vi "Send On Event Message.vi"(8 "error in (no error)":errorcluster, 10 "Event":string, 11 "Observable Actor in":refnum<class "Observable Actor.lvclass">) -> (0 "error out":errorcluster, 3 "Observable Actor out":refnum<class "Observable Actor.lvclass">)   [LabVIEW 2014, in "Observable Actor.lvlib" / "Observable Actor.lvclass"]
uses:
  Observable Actor.lvclass
  Observable Actor.lvclass/Observable Actor.ctl
  <vilib>/ActorFramework/Message Enqueuer/Message Enqueuer.lvclass/Message Enqueuer.ctl
  <vilib>/ActorFramework/Message Priority Queue/Priority Enqueue.vi
  <vilib>/ActorFramework/Message Enqueuer/Message Enqueuer.lvclass
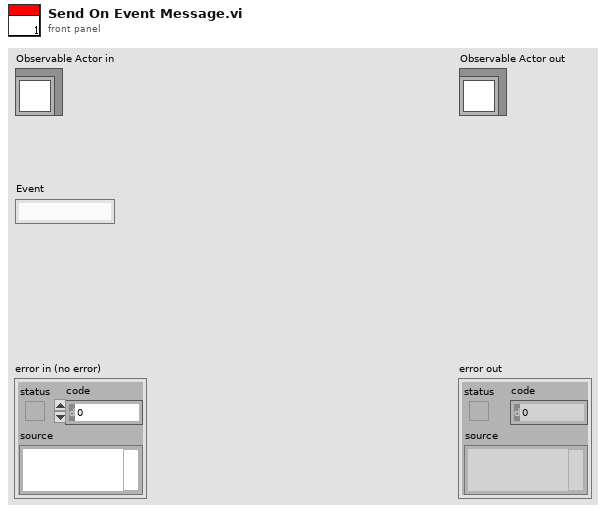
[diagram p1: front panel]
types:
  T1 = typedef "MessageToSend.ctl" = cluster{"Enqueuer":refnum<class "Message Enqueuer.lvclass">, "Message":refnum<class "Message.lvclass">}
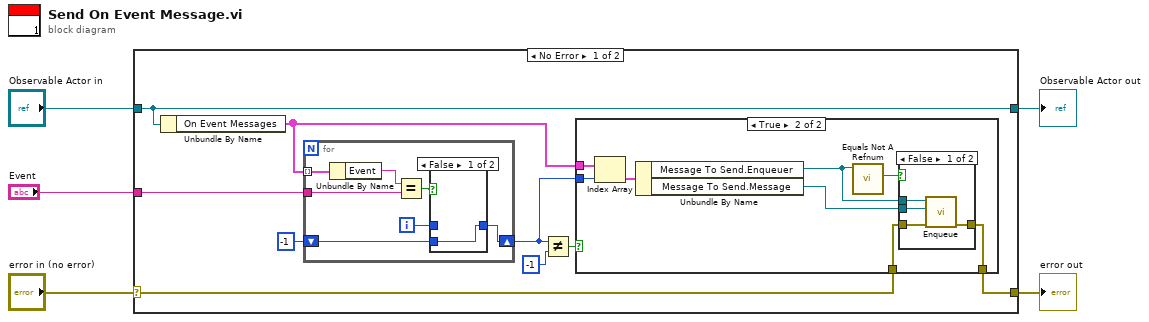
[diagram p0: block diagram]
diagram:
  n1 = case shown="No Error" "error in (no error)" {
    selector: "error in (no error)" -> [w7 w39]
    tunnel: [w6 w39] -> w4
    tunnel: [w14 w38] -> w2
    tunnel: "Observable Actor in" -> [w14 w38]
    tunnel: "Event" -> [w13 _]
    frame No Error {
      n2 = Unbundle By Name(w14) -> ("On Event Messages"=w9:cluster{"Event":string, "Message To Send":T1}[])
      n3 = for {
        tunnel: w9 -> [w35] mode=indexing
        tunnel: w13 -> [w32]
        shift-right: [w30] -> w8
        shift-left: -1 -> [w29]
        i -> [w31]
        n4 = Unbundle By Name(w35) -> ("Event"=w33:string)
        n5 = Equal?(x=w33, y=w32) -> (x = y?=w34:bool)
        n6 = case shown="False" w34 {
          tunnel: w31 -> [_ w37]
          tunnel: [w36 w37] -> w30
          tunnel: w29 -> [w36 _]
          frame False {
          }
          frame True {
          }
        }
      }
      n7 = Not Equal?(x=w8, y=-1) -> (x != y?=w10:bool)
      n8 = case shown="True" w10 {
        tunnel: w9 -> [_ w23]
        tunnel: w8 -> [_ w22]
        tunnel: w7 -> [w15 w17]
        tunnel: [w15 w16] -> w6
        frame False {
        }
        frame True {
          n9 = Index Array(array=w23, index=w22) -> (element=w21:cluster{"Event":string, "Message To Send":T1})
          n10 = Unbundle By Name(w21) -> ("Message To Send.Enqueuer"=w19:refnum<class "Message Enqueuer.lvclass">, "Message To Send.Message"=w18:refnum<class "Message.lvclass">)
          n11 = call <vilib>:"Equals Not A Refnum.vi"("Message Enqueuer"=w19) -> ("Not a refnum?"=w20:bool)  [unwired: 10 in]
          n12 = case shown="False" w20 {
            tunnel: w18 -> [w26 _]
            tunnel: w19 -> [w27 _]
            tunnel: w17 -> [w25 w28]
            tunnel: [w24 w28] -> w16
            frame False {
              n13 = call <vilib>:"Enqueue.vi"("error in (no error)"=w25, "Message"=w26, "Message Enqueuer in"=w27) -> ("error out"=w24:errorcluster)  [unwired: 7 in, 1 out]
            }
            frame True {
            }
          }
        }
      }
    }
    frame Error {
    }
  }
  "error out" <- w4
  "Observable Actor out" <- w2
